vi "GetCommand _Initialise LCR_.vi"(0 "object in":refnum<class "WK6440B.lvclass">, 5 "error in (no error)":errorcluster) -> (14 "object out":refnum<class "WK6440B.lvclass">, 15 "Command _Initialise LCR_":string, 19 "error out":errorcluster)   [LabVIEW 2013, in "WK6440B.lvclass"]
uses:
  WK6440B.lvclass
  WK6440B.lvclass/WK6440B.ctl
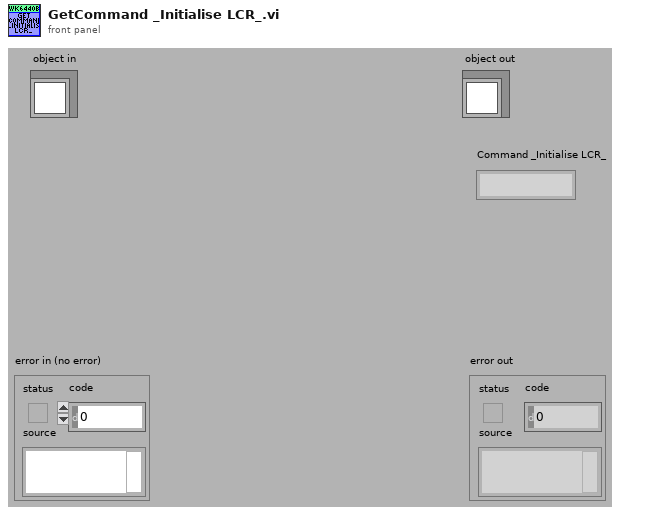
[diagram p1: front panel]
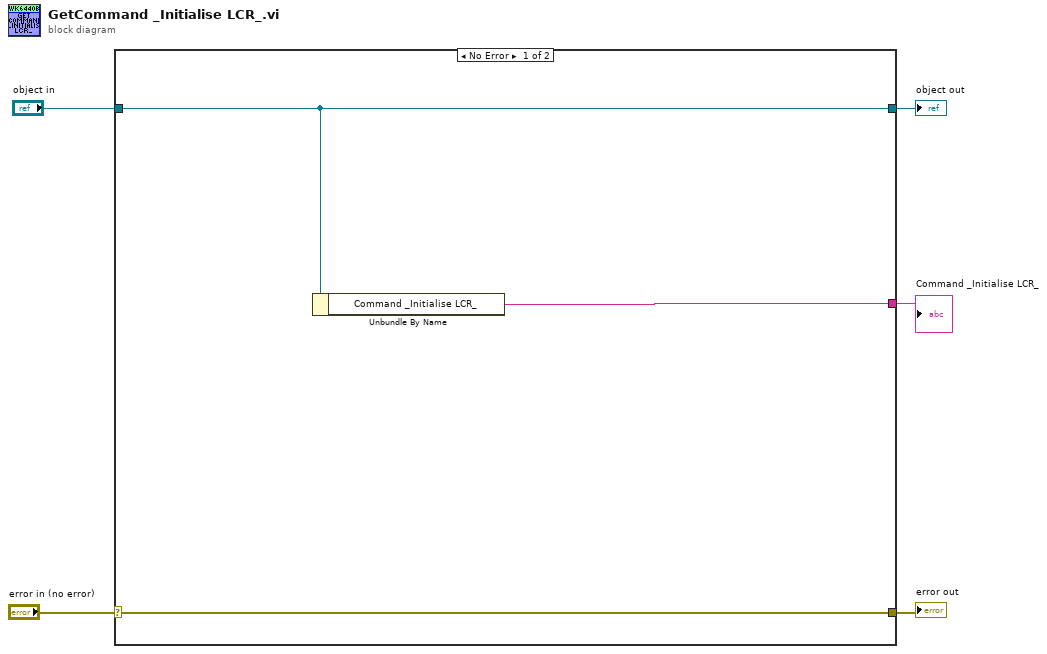
[diagram p0: block diagram]
diagram:
  n1 = case shown="No Error" "error in (no error)" {
    selector: "error in (no error)" -> [w7 w10]
    tunnel: [w7 w10] -> w4
    tunnel: [w6 w9] -> w2
    tunnel: "object in" -> [w6 w9]
    tunnel: [w8 _] -> w1
    frame No Error {
      n2 = Unbundle By Name(w6) -> ("Command _Initialise LCR_"=w8:string)
    }
    frame Error {
    }
  }
  "error out" <- w4
  "object out" <- w2
  "Command _Initialise LCR_" <- w1
